vi "PH_Calorimeter_USB.Calc Energy.vi"(1 "Time scale [s]":dbl[](array[numeric]) format="%.2f", 2 "Data without Offset":sgl[](array[numeric]) format="%.2f", 3 "T 1/E [s]":dbl=1.0 format="%.2f", 4 "sensitivity":dbl=1.0 format="%.10f", 5 "Output Rate [Hz]":i32) -> (17 "Energy [J]":dbl format="%.8f")   [LabVIEW 2014, in "PH_Calorimeter_USB.lvlib"]
doc: "This VI calculates the energy"
uses:
  PH_Calorimeter_USB.lvlib
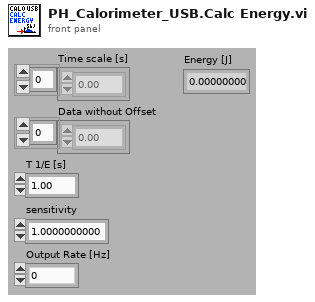
[diagram p1: front panel]
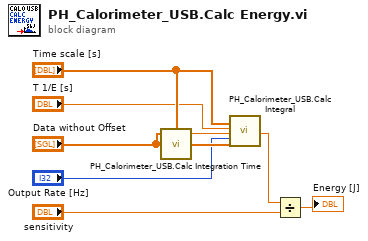
[diagram p0: block diagram]
diagram:
  n1 = call "PH_Calorimeter_USB.Calc Integration Time.vi"("Data without Offset"="Data without Offset", "Time scale [s]"="Time scale [s]") -> ("Integration Time [s]"=w2:dbl)  [unwired: 2 in]
  n2 = call "PH_Calorimeter_USB.Calc Integral.vi"("Time scale [s]"="Time scale [s]", "T 1/E [s]"="T 1/E [s]", "Integration Time [s]"=w2, "Sample Rate [Hz]"="Output Rate [Hz]", "Data without Offset"="Data without Offset") -> ("Integral value"=w1:dbl)  [unwired: 14 in]
  n3 = Divide(x=w1, y="sensitivity") -> (x/y=→"Energy [J]":dbl)
